vi "newValueStep.vi"(8 "error in (no error)":errorcluster, 11 "RampAction in":refnum<class "RampAction.lvclass">) -> (0 "error out":errorcluster, 3 "RampAction out":refnum<class "RampAction.lvclass">)   [LabVIEW 2011, in "Views.lvlib" / "ScriptEditor.lvlib" / "RampAction.lvclass"]
uses:
  RampAction.lvclass
  RampAction.lvclass/RampAction.ctl
  Tools/Scripting/ScriptingEvent/ScriptEvents/Ramp/RampEvent/RampEvent.lvclass
  ActionPanel.lvclass
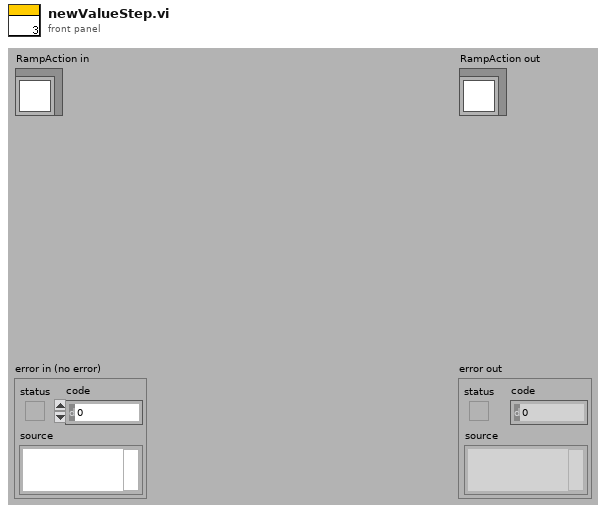
[diagram p1: front panel]
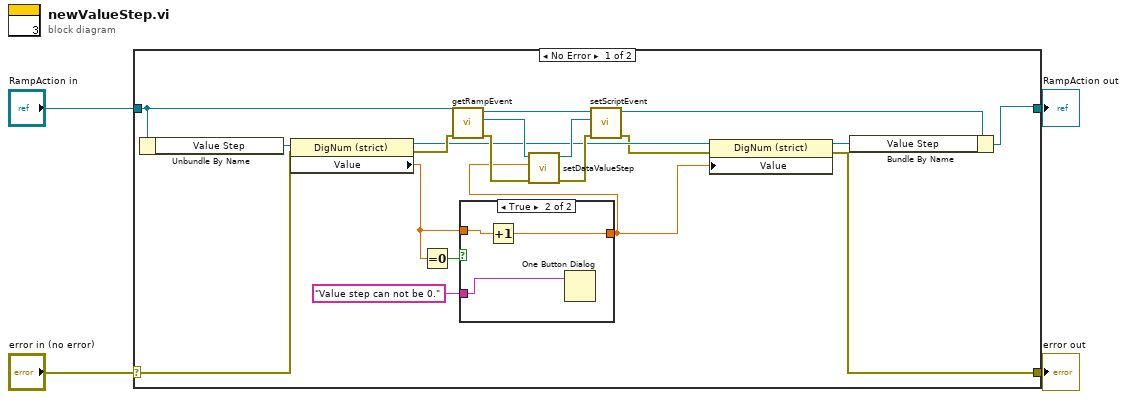
[diagram p0: block diagram]
diagram:
  n1 = case shown="No Error" "error in (no error)" {
    selector: "error in (no error)" -> [w22 w29]
    tunnel: [w6 w29] -> w3
    tunnel: [w12 w28] -> w1
    tunnel: "RampAction in" -> [w21 w28]
    frame No Error {
      n2 = Unbundle By Name(w21) -> ("Value Step"=w23:refnum<vi>)
      n3 = property class="DigNum (strict)"(reference=w23, error in=w22) -> (reference out=w14:refnum<vi>, error out=w20:errorcluster, "Value"=w10:dbl)
      n4 = Equal To 0?(x=w10) -> (x = 0?=w11:bool)
      n5 = call "getRampEvent.vi"("error in (no error)"=w20, "RampAction in"=w21) -> ("error out"=w18:errorcluster, "RampEvent"=w19:refnum<class "RampEvent.lvclass">, "RampAction out"=w17:refnum<class "RampAction.lvclass">)  [unwired: 7 in]
      n6 = case shown="True" w11 {
        tunnel: w10 -> [w24 w27]
        tunnel: [w24 w26] -> w5
        tunnel: "Value step can not be 0." -> [_ w25]
        frame False {
        }
        frame True {
          n7 = Increment(x=w27) -> (x+1=w26:dbl)
          n8 = One Button Dialog(message=w25) -> ()  [unwired: 1 in, 1 out]
        }
      }
      n9 = call "setDataValueStep.vi"("error in (no error)"=w18, "dataValueStep"=w5, "RampEvent.lvclass in"=w19) -> ("error out"=w15:errorcluster, "RampEvent.lvclass out"=w16:refnum<class "RampEvent.lvclass">)  [unwired: 7 in]
      n10 = call "setScriptEvent.vi"("error in (no error)"=w15, "ScriptEvent.lvclass"=w16, "ActionPanel.lvclass in"=w17) -> ("error out"=w7:errorcluster, "ActionPanel.lvclass out"=w13:refnum<class "RampAction.lvclass">)  [unwired: 7 in]
      n11 = property class="DigNum (strict)"(reference=w14, error in=w7, "Value"=w5) -> (reference out=w8:refnum<vi>, error out=w6:errorcluster)
      n12 = Bundle By Name(cluster=w13, "Value Step"=w8) -> (w12:refnum<class "RampAction.lvclass">)
    }
    frame Error {
    }
  }
  "error out" <- w3
  "RampAction out" <- w1
